vi "Set Carrier Phase.vi"(0 "Session Handle in":T1, 5 "Phase":dbl, 11 "error in (no error)":errorcluster) -> (4 "Session Handle out":T1, 6 "Error Code":string, 15 "error out":errorcluster)   [LabVIEW 2015, in "PAS.lvclass"]
uses:
  PAS.lvclass
  Typedefs/Session Handle.ctl
panel:
  out "Success?":bool
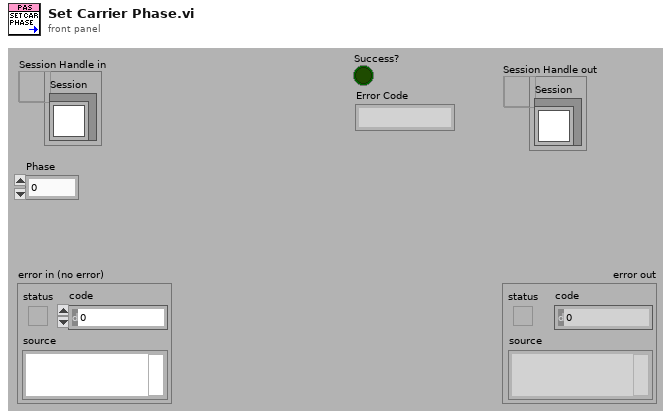
[diagram p1: front panel]
types:
  T1 = typedef "PAS.lvclass/Session Handle.ctl" = refnum<data-value>
  T2 = typedef "XNET Frame CAN.ctl" = cluster{"timestamp":timestamp, "payload":u8[], "identifier":u32, "type":T3, "extended?":bool, "echo?":bool}
  T3 = typedef "XNET Frame Type CAN.ctl" = u8
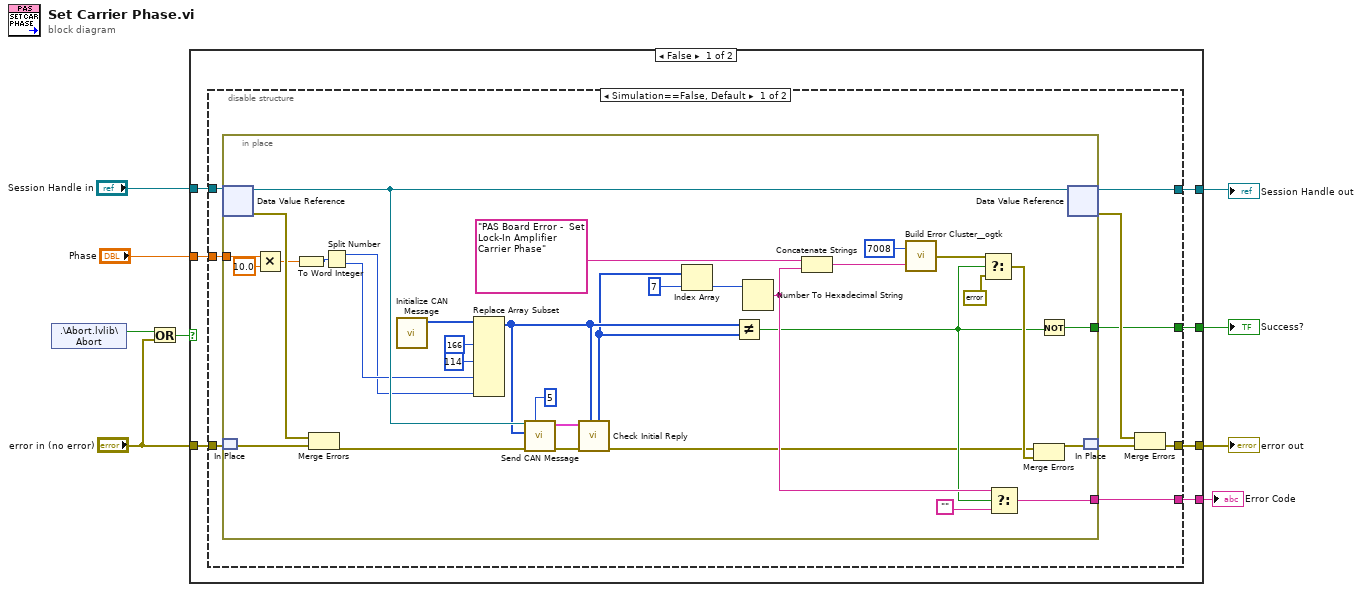
[diagram p0: block diagram]
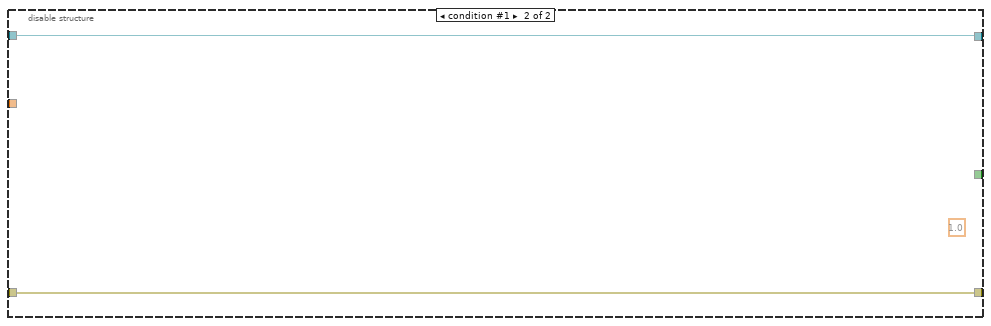
[diagram p2: hidden frame]
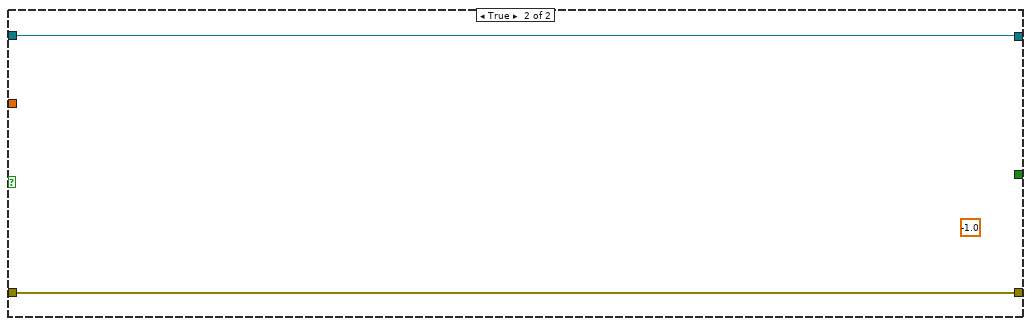
[diagram p3: hidden frame]
diagram:
  n1 = shared-variable ".\\Abort.lvlib\\Abort"() -> (w6:bool)  [unwired: 1 in, 1 out]
  n2 = Or(x=w6, y="error in (no error)") -> (x .or. y?=w4:bool)
  n3 = case shown="False" w4 {
    tunnel: [w16 w62] -> w8
    tunnel: [w15 w61] -> w7
    tunnel: "Session Handle in" -> [w14 w62]
    tunnel: "error in (no error)" -> [w13 w61]
    tunnel: [w12 _] -> w3
    tunnel: "Phase" -> [w11 _]
    tunnel: [w10 _] -> w1
    frame False {
      n4 = disable-structure shown="Simulation==False, Default" {
        disable-tunnel: [w25 w60] -> w16
        disable-tunnel: [w22 w59] -> w15
        disable-tunnel: w14 -> [w21 w60]
        disable-tunnel: w13 -> [w20 w59]
        disable-tunnel: [w19 _] -> w12
        disable-tunnel: w11 -> [w18 _]
        disable-tunnel: [w17 _] -> w10
        frame condition #0 (active) {
          n5 = in-place {
            in-place-border: [w48] -> w19
            in-place-border: w18 -> [w40]
            in-place-border: [w28] -> w17
            n6 = in-place-dvr #1(w21) -> (w51:refnum<class "PAS.lvclass">, w55:errorcluster)
            n7 = in-place-match #2(w20) -> (w54:errorcluster)
            n8 = Multiply(x=w40, y=10.0) -> (x*y=w38:dbl)
            n9 = To Word Integer(number=w38) -> (16bit integer=w43:i16)
            n10 = Merge Errors(w55, w54) -> (w50:errorcluster)
            n11 = Split Number(x=w43) -> (hi(x)=w41:u8, lo(x)=w42:u8)
            n12 = call "Initialize CAN Message.vi"() -> ("Initial Payload"=w56:u8[])  [unwired: 11 in]
            n13 = Replace Array Subset(array=w56, new element #1=u8 166 ("new element/subarray"), new element #2=u8 114 ("new element/subarray"), new element #3=w42, new element #4=w41) -> (w37:u8[])  [unwired: 4 in]
            n14 = call "Send CAN Message.vi"("Number of Retries"=5, "error in (no error)"=w50, "payload"=w37, "Gas In"=w51) -> ("error out"=w27:errorcluster, "Reply"=w52:T2[])  [unwired: 5 in, 1 out]
            n15 = call "Check Initial Reply.vi"("Write Message"=w37, "error in (no error)"=w27, "Reply"=w52) -> ("error out"=w26:errorcluster, "Whole Payload"=w33:u8[])  [unwired: 5 in, 2 out]
            n16 = Index Array(array=w33, index=7) -> (element=w35:u8)
            n17 = Not Equal?(x=w37, y=w33) -> (x != y?=w29:bool)
            n18 = Number To Hexadecimal String(2:w35) -> (0:w30:string)  [unwired: 1 in]
            n19 = Concatenate Strings("PAS Board Error -  Set Lock-In Amplifier Carrier Phase" ("string"), w30) -> (w34:string)
            n20 = call <userlib>:"Build Error Cluster__ogtk.vi"("String to Prepend to source (\"\")"=w34, "code"=7008) -> ("error out"=w47:errorcluster)
            n21 = Select(t=w47, s=w29, f=errorcluster {"status"=FALSE, "code"=0, "source"=""}) -> (s? t:f=w44:errorcluster)
            n22 = Select(t=w30, s=w29, f="") -> (s? t:f=w28:string)
            n23 = Merge Errors(w26, w44) -> (w57:errorcluster)
            n24 = Not(x=w29) -> (.not. x?=w48:bool)
            n25 = in-place-dvr #1(w51) -> (w25:T1, w23:errorcluster)
            n26 = in-place-match #2(w57) -> (w24:errorcluster)
          }
          n27 = Merge Errors(w23, w24) -> (w22:errorcluster)
        }
        frame condition #1 {
          (unwired) 1.0
        }
      }
    }
    frame True {
      (unwired) -1.0
    }
  }
  "Session Handle out" <- w8
  "error out" <- w7
  "Success?" <- w3
  "Error Code" <- w1
